vi "QuickImageClusterIni.vi"(0 "lines":u32, 1 "planes":u32, 2 "No. of Channels":u16, 3 "pixel per line":u32, 4 "48bit?":bool) -> (5 "IMAGE Cluster":T1)   [LabVIEW 2009]
uses:
  ImageCluster.ctl
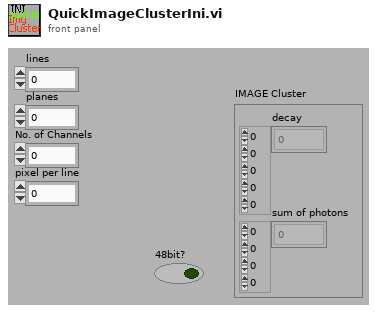
[diagram p1: front panel]
types:
  T1 = typedef "ImageCluster.ctl" = cluster{"decay":u16[][][][][], "sum of photons":u32[][][][]}
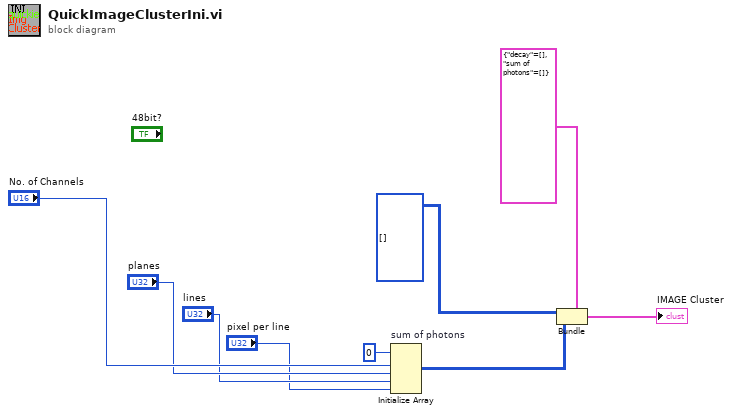
[diagram p0: block diagram]
diagram:
  n1 = Initialize Array "sum of photons"(u32 0 ("element"), "No. of Channels", "planes", "lines", "pixel per line") -> (w9:u32[][][][])
  n2 = Bundle(cluster=T1 {"decay"=[], "sum of photons"=[]} ("IMAGE Cluster 2"), "decay"=u16[][][][][] [], "sum of photons"=w9) -> (→"IMAGE Cluster":T1)
